vi "Find Clones.vi"(7 "Search Clones Up To":i32=100, 10 "VIs in":string[](array[string]), 11 "Application in":refnum<vi>) -> (2 "VIs (including clones) out":string[](array[string]))   [LabVIEW 2013]
doc: "Given a list of VIs in memory, and belonging to a particular Application Instance; this VI returns the input list, plus up to N instances of all statically-referenced AND dynamically-referenced clones currently in memory. All clones are enumerated."
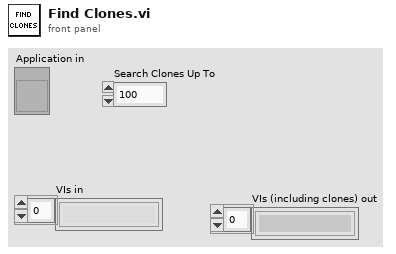
[diagram p1: front panel]
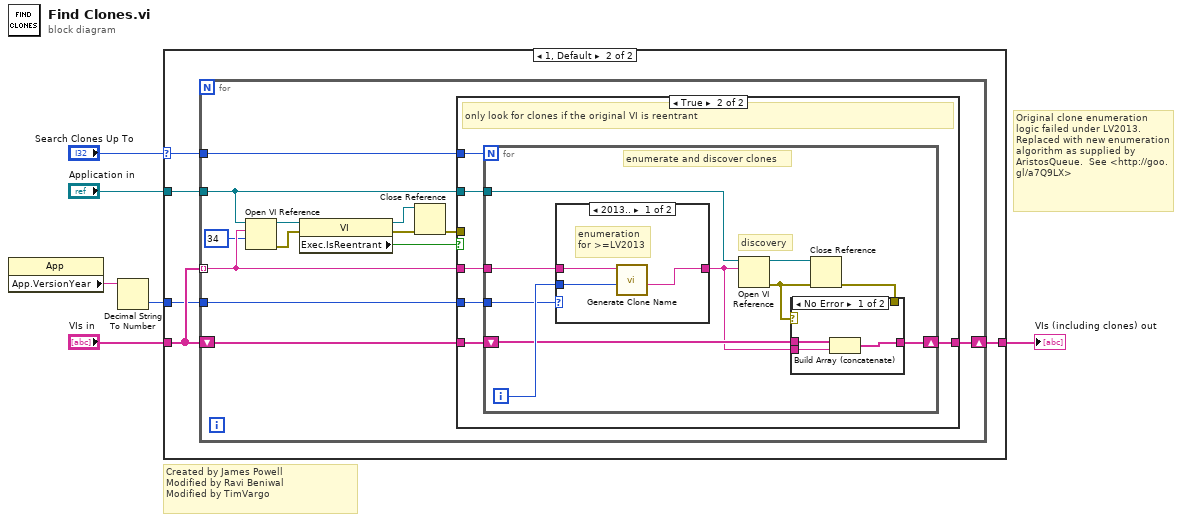
[diagram p0: block diagram]
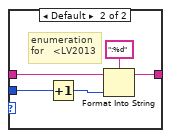
[diagram p4: hidden frame]
diagram:
  # "Original clone enumeration logic failed under LV2013.  Replaced with new enumeration algorithm as supplied by AristosQueue.  See <http://goo.gl/a7Q9LX>"
  # "Created by James Powell\nModified by Ravi Beniwal\nModified by TimVargo"
  n1 = property class="App"() -> ("App.VersionYear"=w2:string)  [unwired: 2 in, 2 out]
  n2 = Decimal String To Number(string=w2) -> (number=w1:i32)  [unwired: 2 in, 1 out]
  n3 = case shown="1, Default" "Search Clones Up To" {
    selector: "Search Clones Up To" -> [_ w9]
    tunnel: [w7 w12] -> w6
    tunnel: "Application in" -> [_ w11]
    tunnel: "VIs in" -> [w7 w10]
    tunnel: w1 -> [_ w8]
    frame 0 {
    }
    frame 1, Default {
      n4 = for {
        tunnel: w10 -> [w19] mode=indexing
        tunnel: w11 -> [w20]
        shift-right: [w18] -> w12
        shift-left: w10 -> [w16]
        tunnel: w9 -> [w17]
        tunnel: w8 -> [w14]
        n5 = Open VI Reference(application reference (local)=w20, vi path=w19, options=34) -> (vi reference=w24:refnum<vi>, error out=w25:errorcluster)  [unwired: 3 in]
        n6 = property class="VI"(reference=w24, error in=w25) -> (reference out=w23:refnum<vi>, error out=w22:errorcluster, "Exec.IsReentrant"=w21:bool)
        n7 = Close Reference(reference=w23, error in (no error)=w22) -> (error out=w15:errorcluster)
        n8 = case shown="True" w21 {
          tunnel: w19 -> [_ w32]
          tunnel: w20 -> [_ w31]
          tunnel: w16 -> [w26 w30]
          tunnel: [w26 w29] -> w18
          tunnel: w17 -> [_ w28]
          tunnel: w15 -> [_ _]
          tunnel: w14 -> [_ w27]
          frame False {
            # "the original VI is not reentrant"
          }
          frame True {
            # "only look for clones if the original VI is reentrant"
            n9 = for {
              N: w28 -> [_]
              tunnel: w32 -> [w42]
              tunnel: w31 -> [w38]
              shift-right: [w40] -> w29
              shift-left: w30 -> [w39]
              tunnel: w27 -> [w33]
              i -> [w41]
              # "discovery"
              # "enumerate and discover clones"
              n10 = case shown="2013.." w33 {
                tunnel: w42 -> [w45 w50]
                tunnel: w41 -> [w44 w49]
                tunnel: [w43 w48] -> w35
                frame 2013.. {
                  # "enumeration\nfor >=LV2013"
                  n11 = call "Generate Clone Name.vi"("Clone number (1)"=w44, "Fully qualified VI name"=w45) -> ("Fully qualified clone name"=w43:string)  [unwired: 7 in, 2 out]
                }
                frame Default {
                  # "enumeration\nfor   <LV2013"
                  n12 = Increment(x=w49) -> (x+1=w46:i32)
                  n13 = Format Into String(format string=":%d", initial string=w50, w46) -> (resulting string=w48:string)  [unwired: 1 in, 1 out]
                }
              }
              n14 = Open VI Reference(application reference (local)=w38, vi path=w35) -> (vi reference=w36:refnum<vi>, error out=w37:errorcluster)  [unwired: 4 in]
              n15 = Close Reference(reference=w36, error in (no error)=w37) -> (error out=w34:errorcluster)
              n16 = case shown="No Error" w37 {
                tunnel: [w53 w54] -> w40
                tunnel: w39 -> [w52 w54]
                tunnel: w35 -> [w51 _]
                tunnel: w34 -> [_ _]
                frame No Error {
                  n17 = Build Array (concatenate)(w52, w51) -> (w53:string[])
                }
                frame Error {
                }
              }
            }
          }
        }
      }
    }
  }
  "VIs (including clones) out" <- w6
